vi "Hatch Panel Intake Global.vi"() -> ()   [LabVIEW 2018]
panel:
  out "Auto Hatch":bool
  out "TeleHatch":bool
  out "Hatch Grab Done":bool=TRUE
  in  "Release Panel":bool
  in  "?":enum16{""}(ring)
  in  "Disable The VI":bool
  in  "Mode":T1(ring)
  in  "State":T2(ring)
  out "Limit Switch":bool
  out "Extended?":bool
  out "Opened?":bool
  out "PanelSensor":bool
  in  "HatchExtend":bool
  in  "HatchGrab":bool
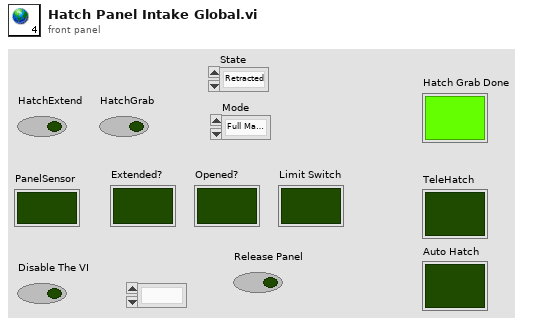
[diagram p1: front panel]
types:
  T1 = enum16{"Full Manual Control", "Manual Control", "Autonomous Control", "Fully Autonomous Control"}
  T2 = enum16{"Retracted", "Extended Open", "Extended Close", "Moving", "Grabbing Hatch Panel", "Placing Hatch Panel"}
diagram:
